vi "Test All.vi"() -> (3 "all_passed":bool)   [LabVIEW 2022 SP3]
doc: "Tests all Hashlib VIs"
panel:
  out "passed":bool[](array[boolean])
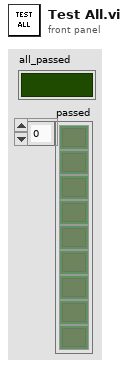
[diagram p1: front panel]
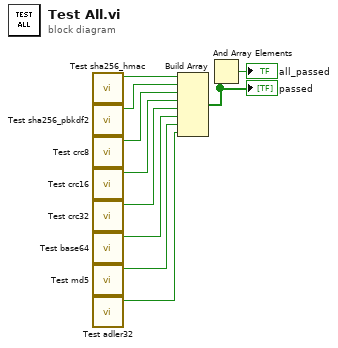
[diagram p0: block diagram]
diagram:
  n1 = call "Test sha256_hmac.vi"() -> ("all_passed"=w9:bool)  [unwired: 11 in]
  n2 = call "Test sha256_pbkdf2.vi"() -> ("all_passed"=w8:bool)  [unwired: 11 in]
  n3 = call "Test crc8.vi"() -> ("All Passed?"=w3:bool)  [unwired: 11 in]
  n4 = call "Test crc16.vi"() -> ("All Passed?"=w6:bool)  [unwired: 11 in]
  n5 = call "Test crc32.vi"() -> ("All Passed?"=w4:bool)  [unwired: 11 in]
  n6 = call "Test base64.vi"() -> ("All Passed?"=w5:bool)  [unwired: 11 in]
  n7 = call "Test md5.vi"() -> ("All Passed?"=w2:bool)  [unwired: 11 in]
  n8 = call "Test adler32.vi"() -> ("All Passed?"=w1:bool)  [unwired: 11 in]
  n9 = Build Array(w9, w8, w3, w6, w4, w5, w2, w1) -> (w7:bool[])
  "passed" <- w7
  n10 = And Array Elements(Boolean array=w7) -> (logical AND=→"all_passed":bool)
